vi "addTimeToPath.vi"(11 "Path":path) -> (2 "Time Path (Path)":path, 3 "Time Path (String)":string)   [LabVIEW 2012]
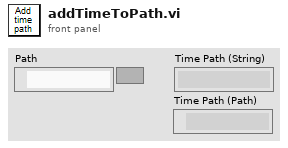
[diagram p1: front panel]
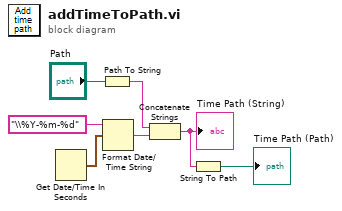
[diagram p0: block diagram]
diagram:
  n1 = Get Date/Time In Seconds() -> (seconds since 1Jan1904=w3:timestamp)
  n2 = Path To String(path="Path") -> (string=w6:string)
  n3 = Format Date/Time String(time format string (%c)="\\%Y-%m-%d", seconds (now)=w3) -> (date/time string=w7:string)  [unwired: 1 in]
  n4 = Concatenate Strings(w6, w7) -> (w2:string)
  "Time Path (String)" <- w2
  n5 = String To Path(string=w2) -> (path=→"Time Path (Path)":path)
